vi "send_data.vi"(7 "Misure":dbl[](array[numeric]), 8 "error in (no error)":errorcluster, 9 "Frequenze":dbl[](array[numeric]), 10 "connection ID in":refnum<k5>, 11 "Digital in":refnum<vi>) -> (0 "error out":errorcluster, 2 "Freq -3dB":dbl, 3 "TCP Network Connection out":refnum<k5>)   [LabVIEW 2021]
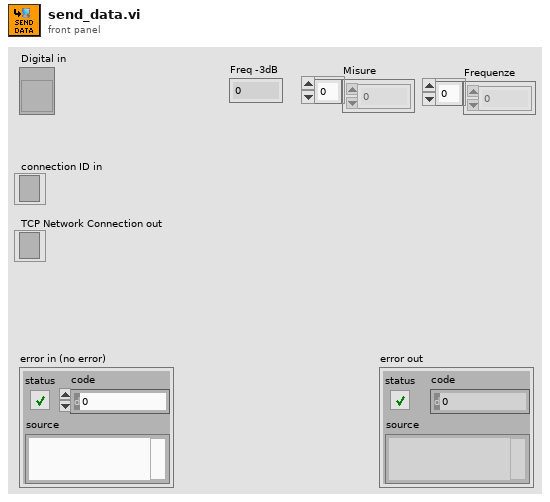
[diagram p1: front panel]
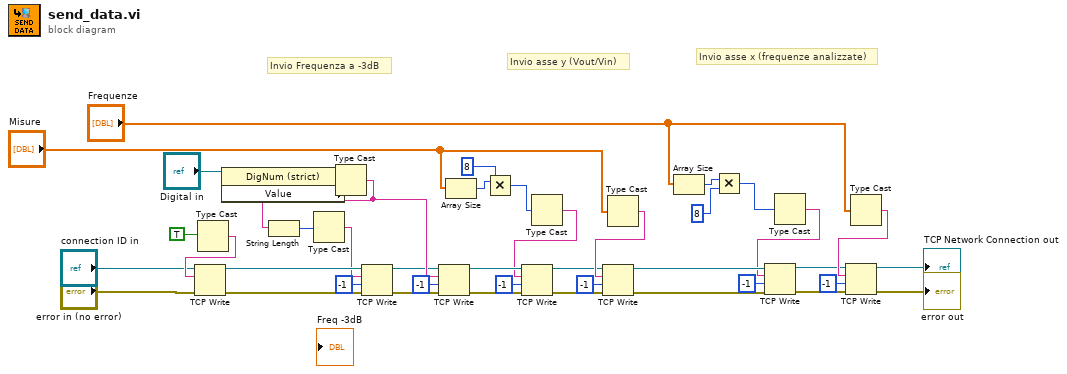
[diagram p0: block diagram]
diagram:
  # "Invio asse x (frequenze analizzate)"
  # "Invio asse y (Vout/Vin)"
  # "Invio Frequenza a -3dB"
  n1 = Type Cast(x=TRUE) -> (*(type *) &x=w4:string)  [unwired: 1 in]
  n2 = TCP Write(connection ID="connection ID in", data in=w4, error in (no error)="error in (no error)") -> (connection ID out=w41:refnum<k5>, error out=w40:errorcluster)  [unwired: 1 in, 1 out]
  n3 = property class="DigNum (strict)"(reference="Digital in") -> ("Value"=w9:dbl)  [unwired: 1 in, 2 out]
  n4 = Type Cast(x=w9) -> (*(type *) &x=w11:string)  [unwired: 1 in]
  n5 = String Length(string=w11) -> (length=w8:i32)
  n6 = Type Cast(x=w8) -> (*(type *) &x=w10:string)  [unwired: 1 in]
  n7 = TCP Write(connection ID=w41, data in=w10, error in (no error)=w40, 9:-1 ("timeout ms (25000)")) -> (connection ID out=w6:refnum<k5>, error out=w7:errorcluster)  [unwired: 1 out]
  n8 = TCP Write(connection ID=w6, data in=w11, error in (no error)=w7, 9:-1 ("timeout ms (25000)")) -> (connection ID out=w17:refnum<k5>, error out=w16:errorcluster)  [unwired: 1 out]
  n9 = Array Size(array="Misure") -> (size(s)=w34:i32)
  n10 = Multiply(x=w34, y=8) -> (x*y=w36:i32)
  n11 = Type Cast(x=w36) -> (*(type *) &x=w12:string)  [unwired: 1 in]
  n12 = TCP Write(connection ID=w17, data in=w12, error in (no error)=w16, 9:-1 ("timeout ms (25000)")) -> (connection ID out=w13:refnum<k5>, error out=w14:errorcluster)  [unwired: 1 out]
  n13 = Type Cast(x="Misure") -> (*(type *) &x=w15:string)  [unwired: 1 in]
  n14 = TCP Write(connection ID=w13, data in=w15, error in (no error)=w14, 9:-1 ("timeout ms (25000)")) -> (connection ID out=w23:refnum<k5>, error out=w24:errorcluster)  [unwired: 1 out]
  n15 = Array Size(array="Frequenze") -> (size(s)=w37:i32)
  n16 = Multiply(x=w37, y=8) -> (x*y=w39:i32)
  n17 = Type Cast(x=w39) -> (*(type *) &x=w19:string)  [unwired: 1 in]
  n18 = TCP Write(connection ID=w23, data in=w19, error in (no error)=w24, 9:-1 ("timeout ms (25000)")) -> (connection ID out=w20:refnum<k5>, error out=w21:errorcluster)  [unwired: 1 out]
  n19 = Type Cast(x="Frequenze") -> (*(type *) &x=w22:string)  [unwired: 1 in]
  n20 = TCP Write(connection ID=w20, data in=w22, error in (no error)=w21, 9:-1 ("timeout ms (25000)")) -> (connection ID out=→"TCP Network Connection out":refnum<k5>, error out=→"error out":errorcluster)  [unwired: 1 out]
